vi "Update VS channels (interaction info).vi"(9 "receiveInteraction in":T1, 10 "hla map helpers in":T6, 11 "values in":dbl[](array[numeric])) -> (1 "receiveInteraction out":T1, 2 "hla map helpers out":T6, 3 "values out":dbl[](array[numeric]))   [LabVIEW 2019, in "HLA Custom Device Engine.lvlib"]
uses:
  HLA Custom Device Engine.lvlib
  RThlaMapHelpers.ctl
  map_interaction.ctl
  map_interaction_value.ctl
  map_attr_param_data.ctl
  map_object.ctl
  map_object_key.ctl
  map_object_value.ctl
  map_object_instance.ctl
  map_object_instance_value.ctl
  receiveInteraction_type.ctl
  interaction_info_received_type.ctl
  emea-ni-adg-hla-lv/src/library/typedefs/TransportationType.ctl
  emea-ni-adg-hla-lv/src/library/typedefs/OrderType.ctl
  dataElement_type.ctl
  emea-ni-adg-hla-lv/src/library/openrti_rti1516eLv.lvlib
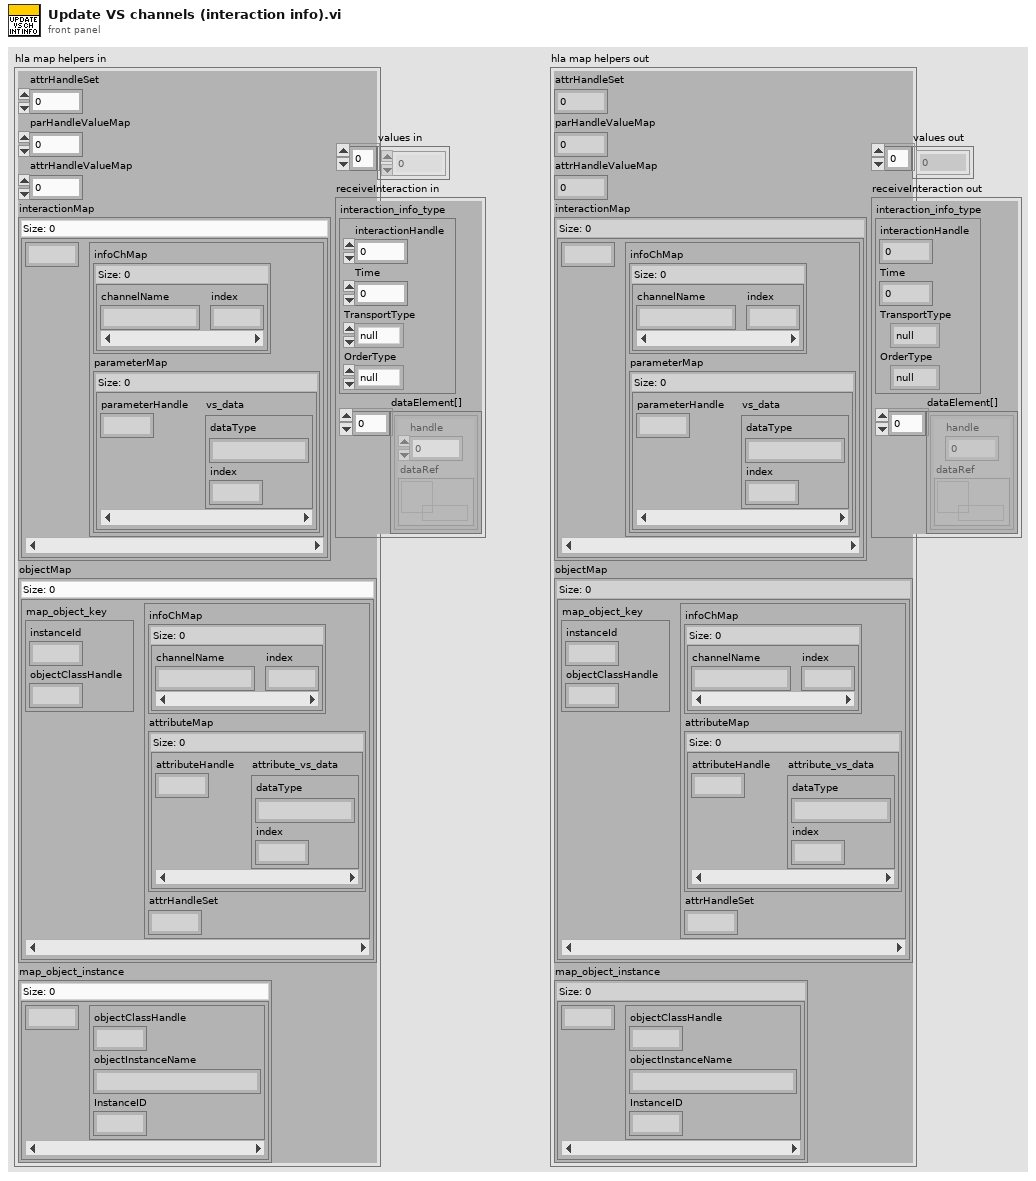
[diagram p1: front panel]
types:
  T1 = typedef "HLA Custom Device Engine.lvlib/receiveInteraction_type.ctl" = cluster{"interaction_info_type":T2, "dataElement[]":T5[]}
  T2 = typedef "HLA Custom Device Engine.lvlib/interaction_info_received_type.ctl" = cluster{"interactionHandle":u64, "Time":u32, "TransportType":T3, "OrderType":T4}
  T3 = typedef "openrti_rti1516eLv.lvlib/TransportationType.ctl" = enum32{"null", "RELIABLE", "BEST_EFFORT"}
  T4 = typedef "openrti_rti1516eLv.lvlib/OrderType.ctl" = enum32{"null", "RECEIVE", "TIMESTAMP"}
  T5 = typedef "HLA Custom Device Engine.lvlib/dataElement_type.ctl" = cluster{"handle":u64, "dataRef":refnum<data-value>}
  T6 = typedef "RThlaMapHelpers.ctl" = cluster{"attrHandleSet":u64, "parHandleValueMap":u64, "attrHandleValueMap":u64, "interactionMap":T7, "objectMap":T10, "map_object_instance":T13}
  T7 = typedef "HLA Custom Device Engine.lvlib/map_interaction.ctl" = map{u64, T8}
  T8 = typedef "HLA Custom Device Engine.lvlib/map_interaction_value.ctl" = cluster{"infoChMap":map{string, i32}, "parameterMap":map{u64, T9}}
  T9 = typedef "HLA Custom Device Engine.lvlib/map_attr_param_data.ctl" = cluster{"dataType":string, "index":i32}
  T10 = typedef "HLA Custom Device Engine.lvlib/map_object.ctl" = map{T11, T12}
  T11 = typedef "HLA Custom Device Engine.lvlib/map_object_key.ctl" = cluster{"instanceId":i32, "objectClassHandle":u64}
  T12 = typedef "HLA Custom Device Engine.lvlib/map_object_value.ctl" = cluster{"infoChMap":map{string, i32}, "attributeMap":map{u64, T9}, "attrHandleSet":u64}
  T13 = typedef "HLA Custom Device Engine.lvlib/map_object_instance.ctl" = map{u64, T14}
  T14 = typedef "HLA Custom Device Engine.lvlib/map_object_instance_value.ctl" = cluster{"objectClassHandle":u64, "objectInstanceName":string, "InstanceID":i32}
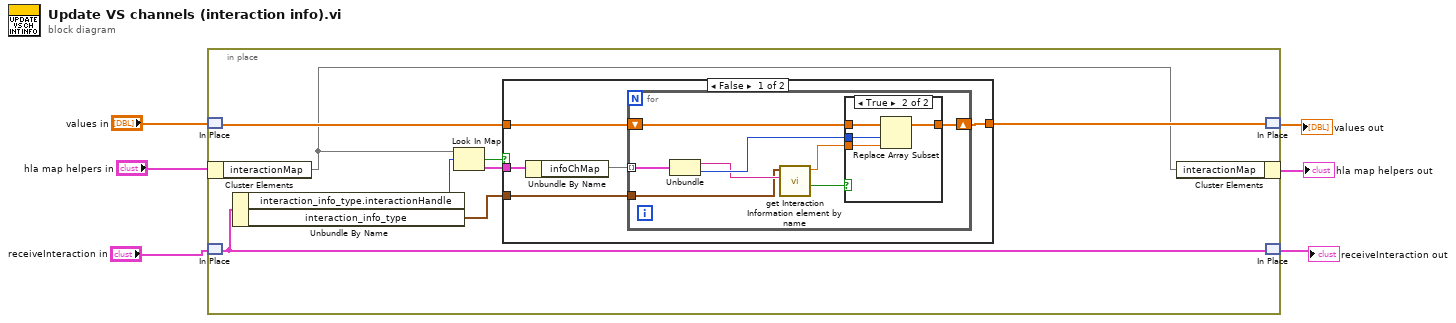
[diagram p0: block diagram]
diagram:
  n1 = in-place {
    n2 = in-place-match #1("values in") -> (w12:dbl[])
    n3 = in-place-cluster #2("hla map helpers in") -> ("interactionMap"=w10:T7)
    n4 = in-place-match #3("receiveInteraction in") -> (w8:T1)
    n5 = Unbundle By Name(w8) -> ("interaction_info_type.interactionHandle"=w9:u64, "interaction_info_type"=w7:T2)
    n6 = Look In Map(map=w10, key=w9) -> (key not found?=w14:bool, value=w13:T8)  [unwired: 1 in]
    n7 = case shown="False" w14 {
      tunnel: [w18 w33] -> w11
      tunnel: w13 -> [w16 _]
      tunnel: w12 -> [w17 w33]
      tunnel: w7 -> [w15 _]
      frame False {
        n8 = Unbundle By Name(w16) -> ("infoChMap"=w19:map{string, i32})
        n9 = for {
          tunnel: w19 -> [w22] mode=indexing
          shift-right: [w26] -> w18
          shift-left: w17 -> [w27]
          tunnel: w15 -> [w20]
          n10 = Unbundle(w22) -> ("channelName"=w21:string, "index"=w24:i32)
          n11 = call "get Interaction Information element by name.vi"("name"=w21, "interaction_attribute_type"=w20) -> ("found"=w23:bool, "element out"=w25:dbl)  [unwired: 8 in]
          n12 = case shown="True" w23 {
            tunnel: w27 -> [w28 w32]
            tunnel: [w28 w31] -> w26
            tunnel: w25 -> [_ w30]
            tunnel: w24 -> [_ w29]
            frame False {
            }
            frame True {
              n13 = Replace Array Subset(array=w32, new element=w30, index=w29) -> (w31:dbl[])
            }
          }
        }
      }
      frame True {
      }
    }
    n14 = in-place-cluster #2("interactionMap"=w10) -> (→"hla map helpers out":T6)
    n15 = in-place-match #1(w11) -> (→"values out":dbl[])
    n16 = in-place-match #3(w8) -> (→"receiveInteraction out":T1)
  }
